vi "Create Pie.vi"(5 "Selection Popout Offset (30)":i16=30, 7 "Rotation Offset (0)":i32, 8 "Colors[] (Use Default)":u32[](array[colorbox]), 9 "Selection (-1)":i32=-1, 10 "Radius":i16, 11 "Values[]":dbl[](array[numeric])) -> (1 "Slice Positions":cluster{"Start":i16, "End":i16}[](array[cluster]), 2 "Pie Draw Area Size":cluster{"Width":i16, "Height":i16}, 3 "Pie out":picture)   [LabVIEW 2018, in "PieChart.lvclass"]
doc: "This method creates the pie portion of the pie chart.\n----\n©2019 Q Software Innovations, LLC\nWritten by Quentin \"Q\" Alldredge\nCLA, LabVIEW Champion"
uses:
  PieChart.lvclass
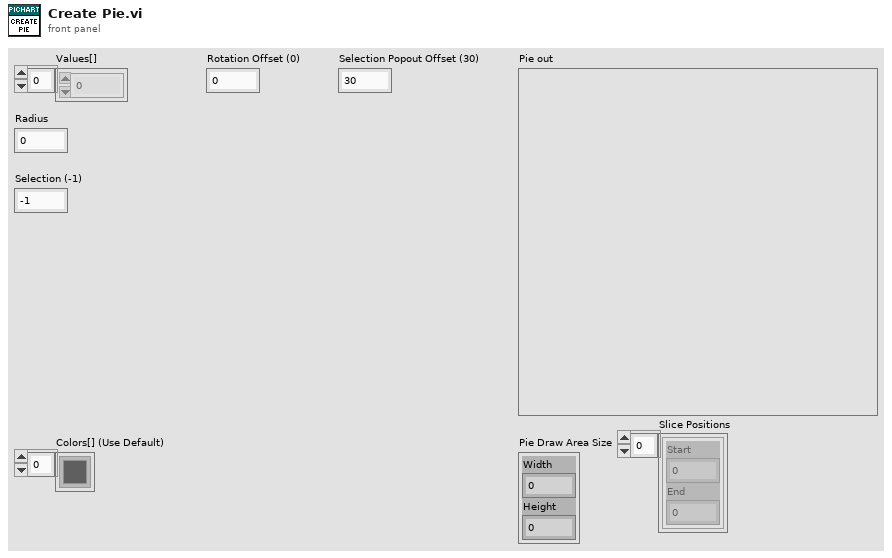
[diagram p1: front panel]
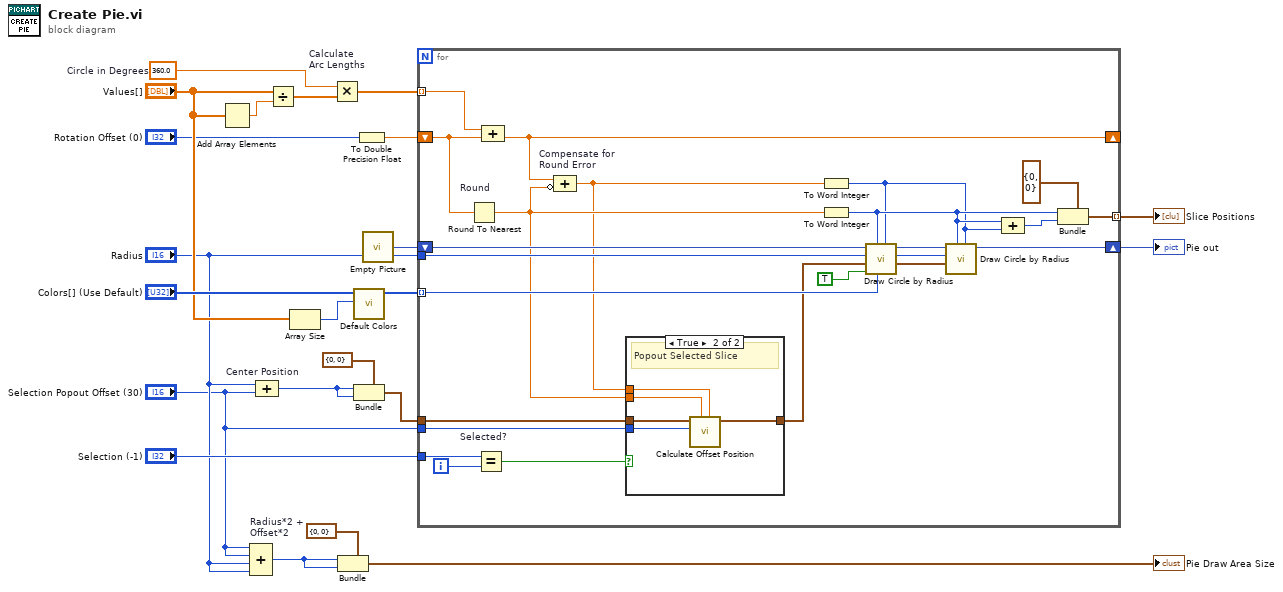
[diagram p0: block diagram]
diagram:
  w20 = 360.0  # Circle in Degrees
  n1 = Add Array Elements(numeric array="Values[]") -> (sum=w22:dbl)
  n2 = Compound Arithmetic op=ADD "Radius*2 +\nOffset*2"("Selection Popout Offset (30)", "Selection Popout Offset (30)", "Radius", "Radius") -> (w3:i16)
  n3 = Compound Arithmetic op=ADD "Center Position"("Radius", "Selection Popout Offset (30)") -> (w10:i16)
  n4 = Divide(x="Values[]", y=w22) -> (x/y=w21:dbl[])
  n5 = Array Size(array="Values[]") -> (size(s)=w13:i32)
  n6 = Multiply "Calculate\nArc Lengths"(x=w20, y=w21) -> (x*y=w17:dbl[])
  n7 = Bundle(cluster=cluster{"Width":i16, "Height":i16} {"Width"=0, "Height"=0} ("Legend Box Size"), "Width"=w3, "Height"=w3) -> (→"Pie Draw Area Size":cluster{"Width":i16, "Height":i16})
  n8 = call "Default Colors.vi"("Number of Entries"=w13, "Colors[] in"="Colors[] (Use Default)") -> ("Colors[] out"=w15:u32[])  [unwired: 9 in]
  n9 = Bundle(cluster=cluster{"horizontal":i16, "vertical":i16} {"horizontal"=0, "vertical"=0} ("pixel center"), "horizontal"=w10, "vertical"=w10) -> (w11:cluster{"horizontal":i16, "vertical":i16})
  n10 = To Double Precision Float(number="Rotation Offset (0)") -> (double precision float=w7:dbl)
  n11 = call "Empty Picture"() -> ("empty picture"=w18:picture)
  n12 = for {
    tunnel: "Radius" -> [w31]
    tunnel: w15 -> [w44] mode=indexing
    shift-right: [w28] -> w12
    shift-left: w18 -> [w42]
    tunnel: w17 -> [w34] mode=indexing
    shift-right: [w32] -> _
    shift-left: w7 -> [w35]
    tunnel: w11 -> [w38]
    tunnel: "Selection (-1)" -> [w40]
    tunnel: "Selection Popout Offset (30)" -> [w37]
    tunnel: [w23] -> w1 mode=indexing
    i -> [w41]
    n13 = Round To Nearest "Round"(number=w35) -> (nearest integer value=w30:dbl)
    n14 = Equal? "Selected?"(x=w40, y=w41) -> (x = y?=w36:bool)
    n15 = Compound Arithmetic op=ADD(w34, w35) -> (w32:dbl)
    n16 = Compound Arithmetic op=ADD "Compensate for \nRound Error"(w32, invert w30) -> (w29:dbl)
    n17 = case shown="True" w36 {
      tunnel: w38 -> [w45 w46]
      tunnel: w37 -> [_ w49]
      tunnel: [w45 w50] -> w33
      tunnel: w30 -> [_ w47]
      tunnel: w29 -> [_ w48]
      frame False {
        # "Draw Normal"
      }
      frame True {
        # "Popout Selected Slice"
        n18 = call "Calculate Offset Position.vi"("Arc Length (degrees)"=w48, "Start Angle (degrees)"=w47, "Offset"=w49, "Original Position"=w46) -> ("Offset Position"=w50:cluster{"horizontal":i16, "vertical":i16})  [unwired: 7 in]
      }
    }
    n19 = To Word Integer(number=w29) -> (16bit integer=w26:i16)
    n20 = To Word Integer(number=w30) -> (16bit integer=w27:i16)
    n21 = call <vilib>:"Draw Circle by Radius.vi"("arc size(360)"=w26, "color(black)"=w44, "start angle(0)"=w27, "fill?(F)"=TRUE, "pixel center"=w33, "radius"=w31, "picture"=w42) -> ("new picture"=w39:picture)  [unwired: 4 in]
    n22 = call <vilib>:"Draw Circle by Radius.vi"("arc size(360)"=w26, "start angle(0)"=w27, "pixel center"=w33, "radius"=w31, "picture"=w39) -> ("new picture"=w28:picture)  [unwired: 6 in]
    n23 = Compound Arithmetic op=ADD(w27, w26) -> (w25:i16)
    n24 = Bundle(cluster=cluster{"Start":i16, "End":i16} {"Start"=0, "End"=0}, "Start"=w27, "End"=w25) -> (w23:cluster{"Start":i16, "End":i16})
  }
  "Pie out" <- w12
  "Slice Positions" <- w1
